vi "Deep Copy.vi"(8 "error in (no error)":errorcluster, 10 "Copy Actor In":refnum<class "System Actor.lvclass">, 11 "System Actor in":refnum<class "System Actor.lvclass">) -> (0 "error out":errorcluster, 2 "Coppied Actor Out":refnum<class "System Actor.lvclass">, 3 "System Actor out":refnum<class "System Actor.lvclass">)   [LabVIEW 2022 SP3, in "System Actor.lvclass"]
uses:
  System Actor.lvclass
  System Actor.lvclass/System Actor.ctl
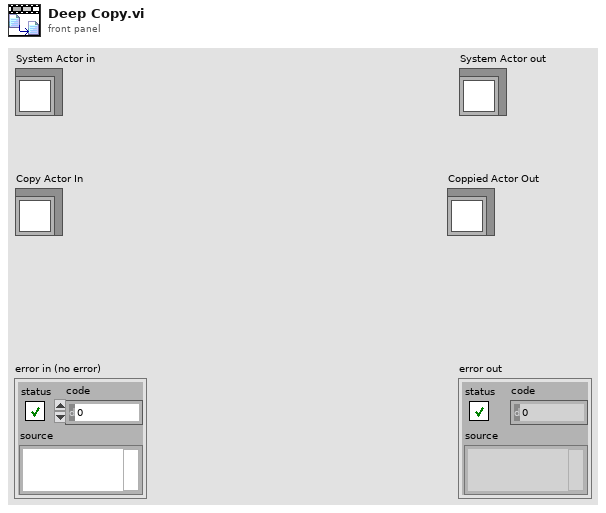
[diagram p1: front panel]
types:
  T1 = typedef "Rendezvous RefNum" = refnum<k1>
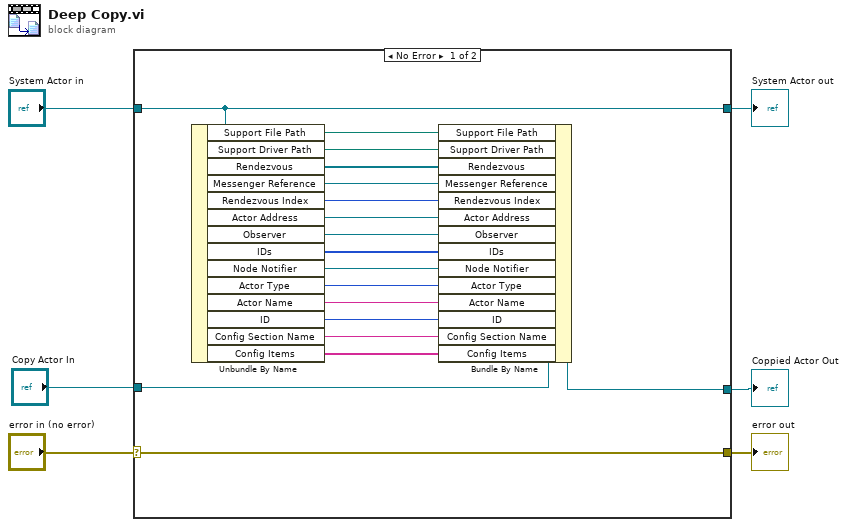
[diagram p0: block diagram]
diagram:
  n1 = case shown="No Error" "error in (no error)" {
    selector: "error in (no error)" -> [w24 w27]
    tunnel: [w24 w27] -> w5
    tunnel: [w23 w26] -> w3
    tunnel: "System Actor in" -> [w23 w26]
    tunnel: "Copy Actor In" -> [w22 w25]
    tunnel: [w7 w25] -> w1
    frame No Error {
      n2 = Unbundle By Name(w23) -> ("Support File Path"=w21:path, "Support Driver Path"=w20:path, "Rendezvous"=w19:T1[], "Messenger Reference"=w18:refnum<data-value>, "Rendezvous Index"=w17:i32, "Actor Address"=w16:refnum<class "Mail Strategy.lvclass">, "Observer"=w15:refnum<class "Observer.lvclass">, "IDs"=w14:i64[], "Node Notifier"=w13:refnum<class "Notifier.lvclass">, "Actor Type"=w12:i64, "Actor Name"=w11:string, "ID"=w10:i64, "Config Section Name"=w9:string, "Config Items"=w8:string[])
      n3 = Bundle By Name(cluster=w22, "Support File Path"=w21, "Support Driver Path"=w20, "Rendezvous"=w19, "Messenger Reference"=w18, "Rendezvous Index"=w17, "Actor Address"=w16, "Observer"=w15, "IDs"=w14, "Node Notifier"=w13, "Actor Type"=w12, "Actor Name"=w11, "ID"=w10, "Config Section Name"=w9, "Config Items"=w8) -> (w7:refnum<class "System Actor.lvclass">)
    }
    frame Error {
    }
  }
  "error out" <- w5
  "System Actor out" <- w3
  "Coppied Actor Out" <- w1
